vi "Error.vi"(8 "Error In":errorcluster, 11 "object in":refnum<class "IStates.lvclass">) -> (0 "Error Out":errorcluster, 3 "object out":refnum<class "IStates.lvclass">)   [LabVIEW 2023, in "HAL.lvlib" / "FGEN.lvlib" / "IStates.lvclass"]
uses:
  IStates.lvclass
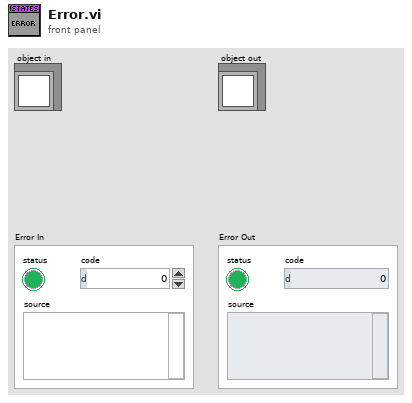
[diagram p1: front panel]
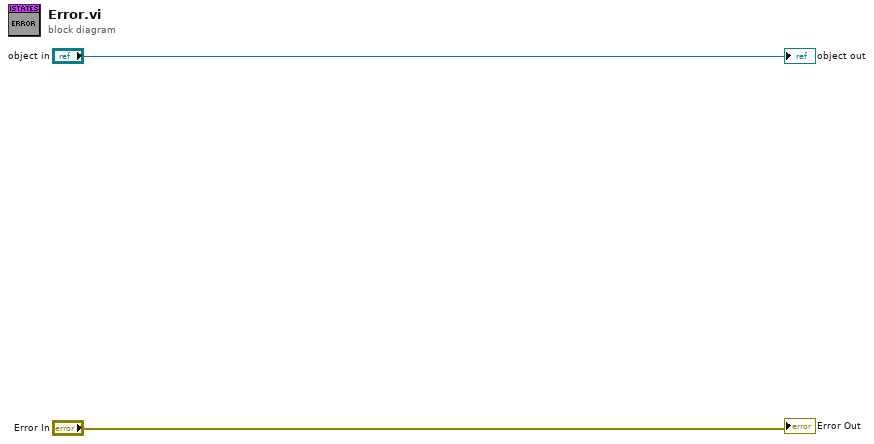
[diagram p0: block diagram]
diagram:
  "Error Out" <- "Error In"
  "object out" <- "object in"
